vi "运维调试_五参数.vi"() -> ()   [LabVIEW 2016, in "斯坦道原位多参数.lvlib"]
uses:
  <vilib>/Utility/miscctls.llb/LVPointTypeDef.ctl
  <vilib>/Utility/config.llb/NI_LVConfig.lvlib
panel:
  in  "校准":bool
  in  "获取传感器参数并保存触发":bool
  in  "传感器参数自动获取":bool=TRUE
  in  "标样测试组数":dbl=1.0 caption="标样测试组数:"
  in  "水样测试组数":dbl=1.0 caption="水样测试组数:"
  in  "转刷清洗时间":dbl=30.0 caption="转刷清洗时间:"
  in  "上电初始化时间":dbl=5.0 caption="上电初始化时间:"
  in  "水样稳定时间":dbl=5.0 caption="水样稳定时间:"
  out "串口号":string
  in  "水深写入":bool
  in  "水深读取":bool
  in  "水深校准":dbl caption="水深校准:"
  out "模块版本号":string
  in  "写入":bool
  in  "读取":bool
  in  "B":dbl caption="校准值B:"
  in  "K":dbl caption="校准值K:"
  in  "标样核查":bool
  in  "串口设置":bool
  in  "质控参数设置":bool
  in  "打开串口":bool
  in  "释放串口":bool
  out "多参数横条运行状态":T1(xcontrol)
  in  "数据区":i32(listbox)
  in  "停止测量(单探)":bool
  in  "启动测量(单探)":bool
  in  "控制命令区探头选择":u16(ring)=9 items=["氨氮"=3, "水温"=9, "pH值"=10, "溶解氧"=11, "电导率"=12, "浊度"=13, "叶绿素a"=14, "藻密度"=15, "蓝绿藻"=16, "氧化还原电位"=17, "溶解氧%"=18, "盐度"=19]
  in  "同步时间":bool
  in  "初始化(清洗)":bool
  in  "停止测量(全部)":bool
  in  "启动测量(全部)":bool
  in  "关键参数区读取":bool
  in  "关键参数区":i32(listbox)
  in  "传感器参数读取":bool
  in  "传感器区":i32(listbox)
  in  "返回":bool
  in  "设置":bool
  out "运行状态":string
  in  "停止":bool
  in  "水样测试":bool
  out "集成报警信息":string
  # "min"
  # "组"
  # "组"
  # "s"
  # "s"
  # "控制命令区"
  # "探头校准"
  # "水深校准"
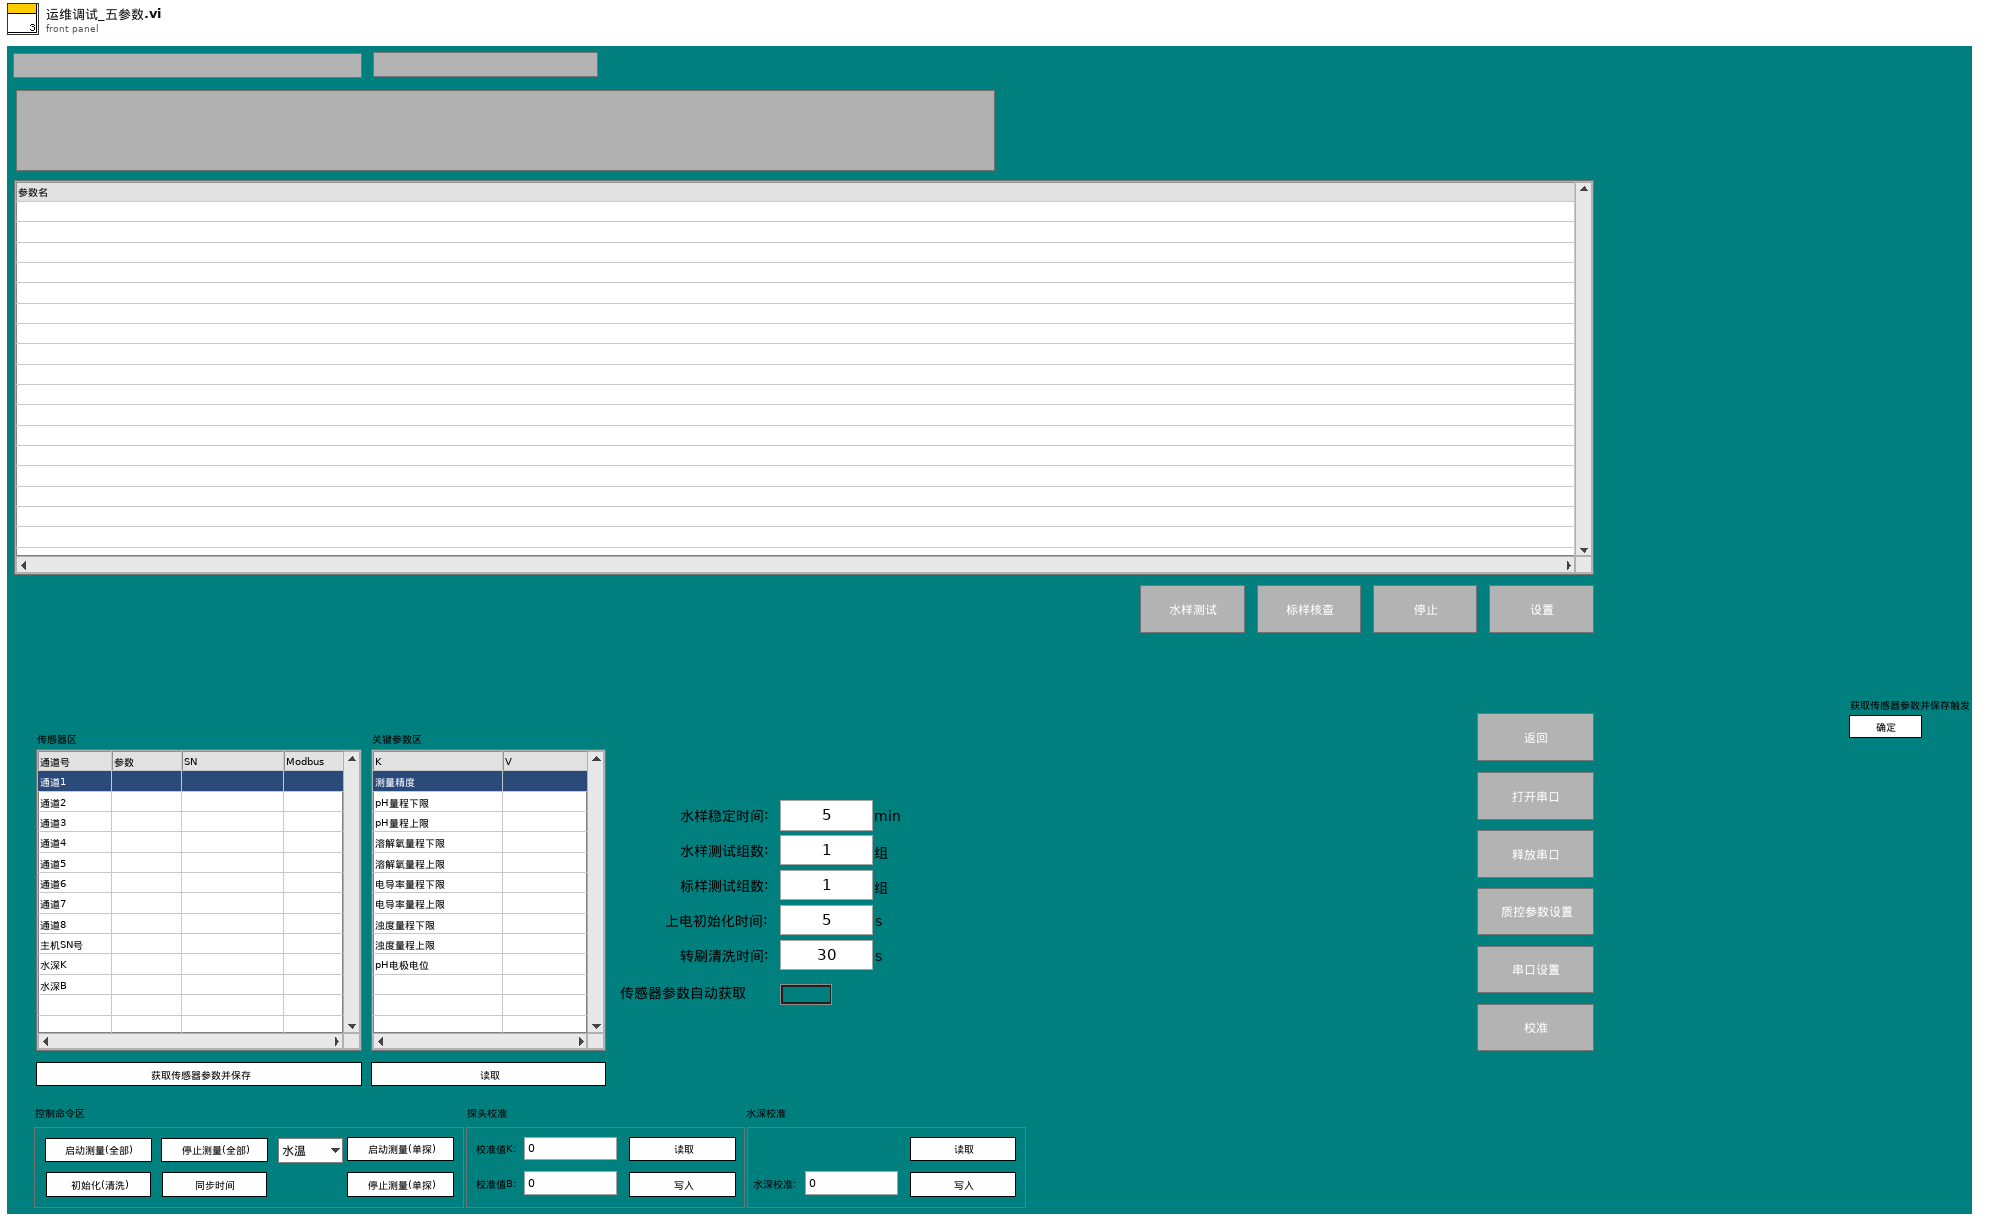
[diagram p1: front panel]
types:
  T1 = cluster{"系统时间":timestamp, "工作状态":u16, "测量模式":u16, "告警代码":enum16{"无告警", "缺试剂告警", "缺水样告警", "缺蒸馏水告警", "缺标液告警", "仪表漏液告警", "标定异常告警", "超量程告警", "加热异常", "低试剂预警", "超上限告警", "超下限告警", "仪表内部其他异常", "滴定异常告警", "电极异常告警", "量程切换告警", "参数设置告警", "PH电极电位异常", "电导率电极异常", "浊度光度异常", "溶解氧电极异常", "溶解氧光强异常", "温度异常告警", "PH异常告警", "溶解氧异常告警", "电导率异常告警", "浊度异常告警", "叶绿素异常告警", "藻密度异常告警", "蓝绿藻异常告警", "ORP异常告警", "氨氮异常告警", "清洁刷异常告警", "SD卡异常告警", "蓝牙异常告警", "Wifi异常告警", "流程异常告警"}, "故障代码":enum16{"无故障", "电机故障", "温度故障", "通讯故障", "滴定故障"}, "日志代码":u16, "软件版本":string}
  T2 = typedef "LVPointTypeDef.ctl" = cluster{"Horizontal":i16, "Vertical":i16}
  T3 = typedef "报警信息字段定义.ctl" = cluster{"时间":timestamp, "参数":string, "报警信息":string, "备注":string, "code":u64, "platform_alarm_code":string}
  T4 = enum16{"无告警", "缺试剂告警", "缺水样告警", "缺蒸馏水告警", "缺标液告警", "仪表漏液告警", "标定异常告警", "超量程告警", "加热异常", "低试剂预警", "超上限告警", "超下限告警", "仪表内部其他异常", "滴定异常告警", "电极异常告警", "量程切换告警", "参数设置告警", "PH电极电位异常", "电导率电极异常", "浊度光度异常", "溶解氧电极异常", "溶解氧光强异常", "温度异常告警", "PH异常告警", "溶解氧异常告警", "电导率异常告警", "浊度异常告警", "叶绿素异常告警", "藻密度异常告警", "蓝绿藻异常告警", "ORP异常告警", "氨氮异常告警", "清洁刷异常告警", "SD卡异常告警", "蓝牙异常告警", "Wifi异常告警", "流程异常告警"}
  T5 = cluster{"水温":dbl, "pH":dbl, "DO":dbl, "Cond":dbl, "Turb":dbl, "叶绿素":dbl, "藻密度":dbl, "蓝绿藻":dbl, "ORP":dbl, "NH3N":dbl}
  T6 = cluster{"因子编码":string, "单位":string, "标样参考值":sgl, "水样数据时间":timestamp, "水样实测值":sgl, "水样数据标识":string, "K":sgl, "B":sgl, "T":sgl, "H":sgl, "水深":sgl, "探头温度":sgl, "信号值":sgl}
  T7 = cluster{"Major":u16, "Minor":u16, "Fix":u16, "Build":u16}
  T8 = enum8{"Enabled", "Disabled", "Disabled and Grayed Out"}
  T9 = typedef "斯坦道原位多参数.lvlib/水样测试启动自定义输入参数.ctl" = cluster{"测量模式":string, "数据类型":string}
  T10 = typedef "斯坦道原位多参数.lvlib/标样核查启动自定义输入参数.ctl" = cluster{"测量模式":string, "数据类型":string, "输出参数":cluster{"水温":bool, "pH":bool, "DO":bool, "浊度":bool, "电导率":bool}}
  T11 = typedef "NI_LVConfig.lvlib/Config Data RefNum.ctl" = refnum<k1>
  T12 = cluster{"水温标准液标准浓度":dbl, "酸碱度标准液标准浓度":dbl, "溶解氧标准液标准浓度":dbl, "电导率标准液标准浓度":dbl, "浊度标准液标准浓度":dbl}
  T13 = cluster{"确定":bool, "水温标准液标准浓度":dbl, "酸碱度标准液标准浓度":dbl, "溶解氧标准液标准浓度":dbl, "电导率标准液标准浓度":dbl, "浊度标准液标准浓度":dbl}
  T14 = cluster{"运行模式":enum16{"维护模式", "常规模式", "应急模式", "质控模式"}, "24H周期设置":bool[]}
  T15 = cluster{"水温":bool, "pH":bool, "DO":bool, "浊度":bool, "电导率":bool}
  T16 = enum32{"Bad", "Idle", "Run top level", "Running"}
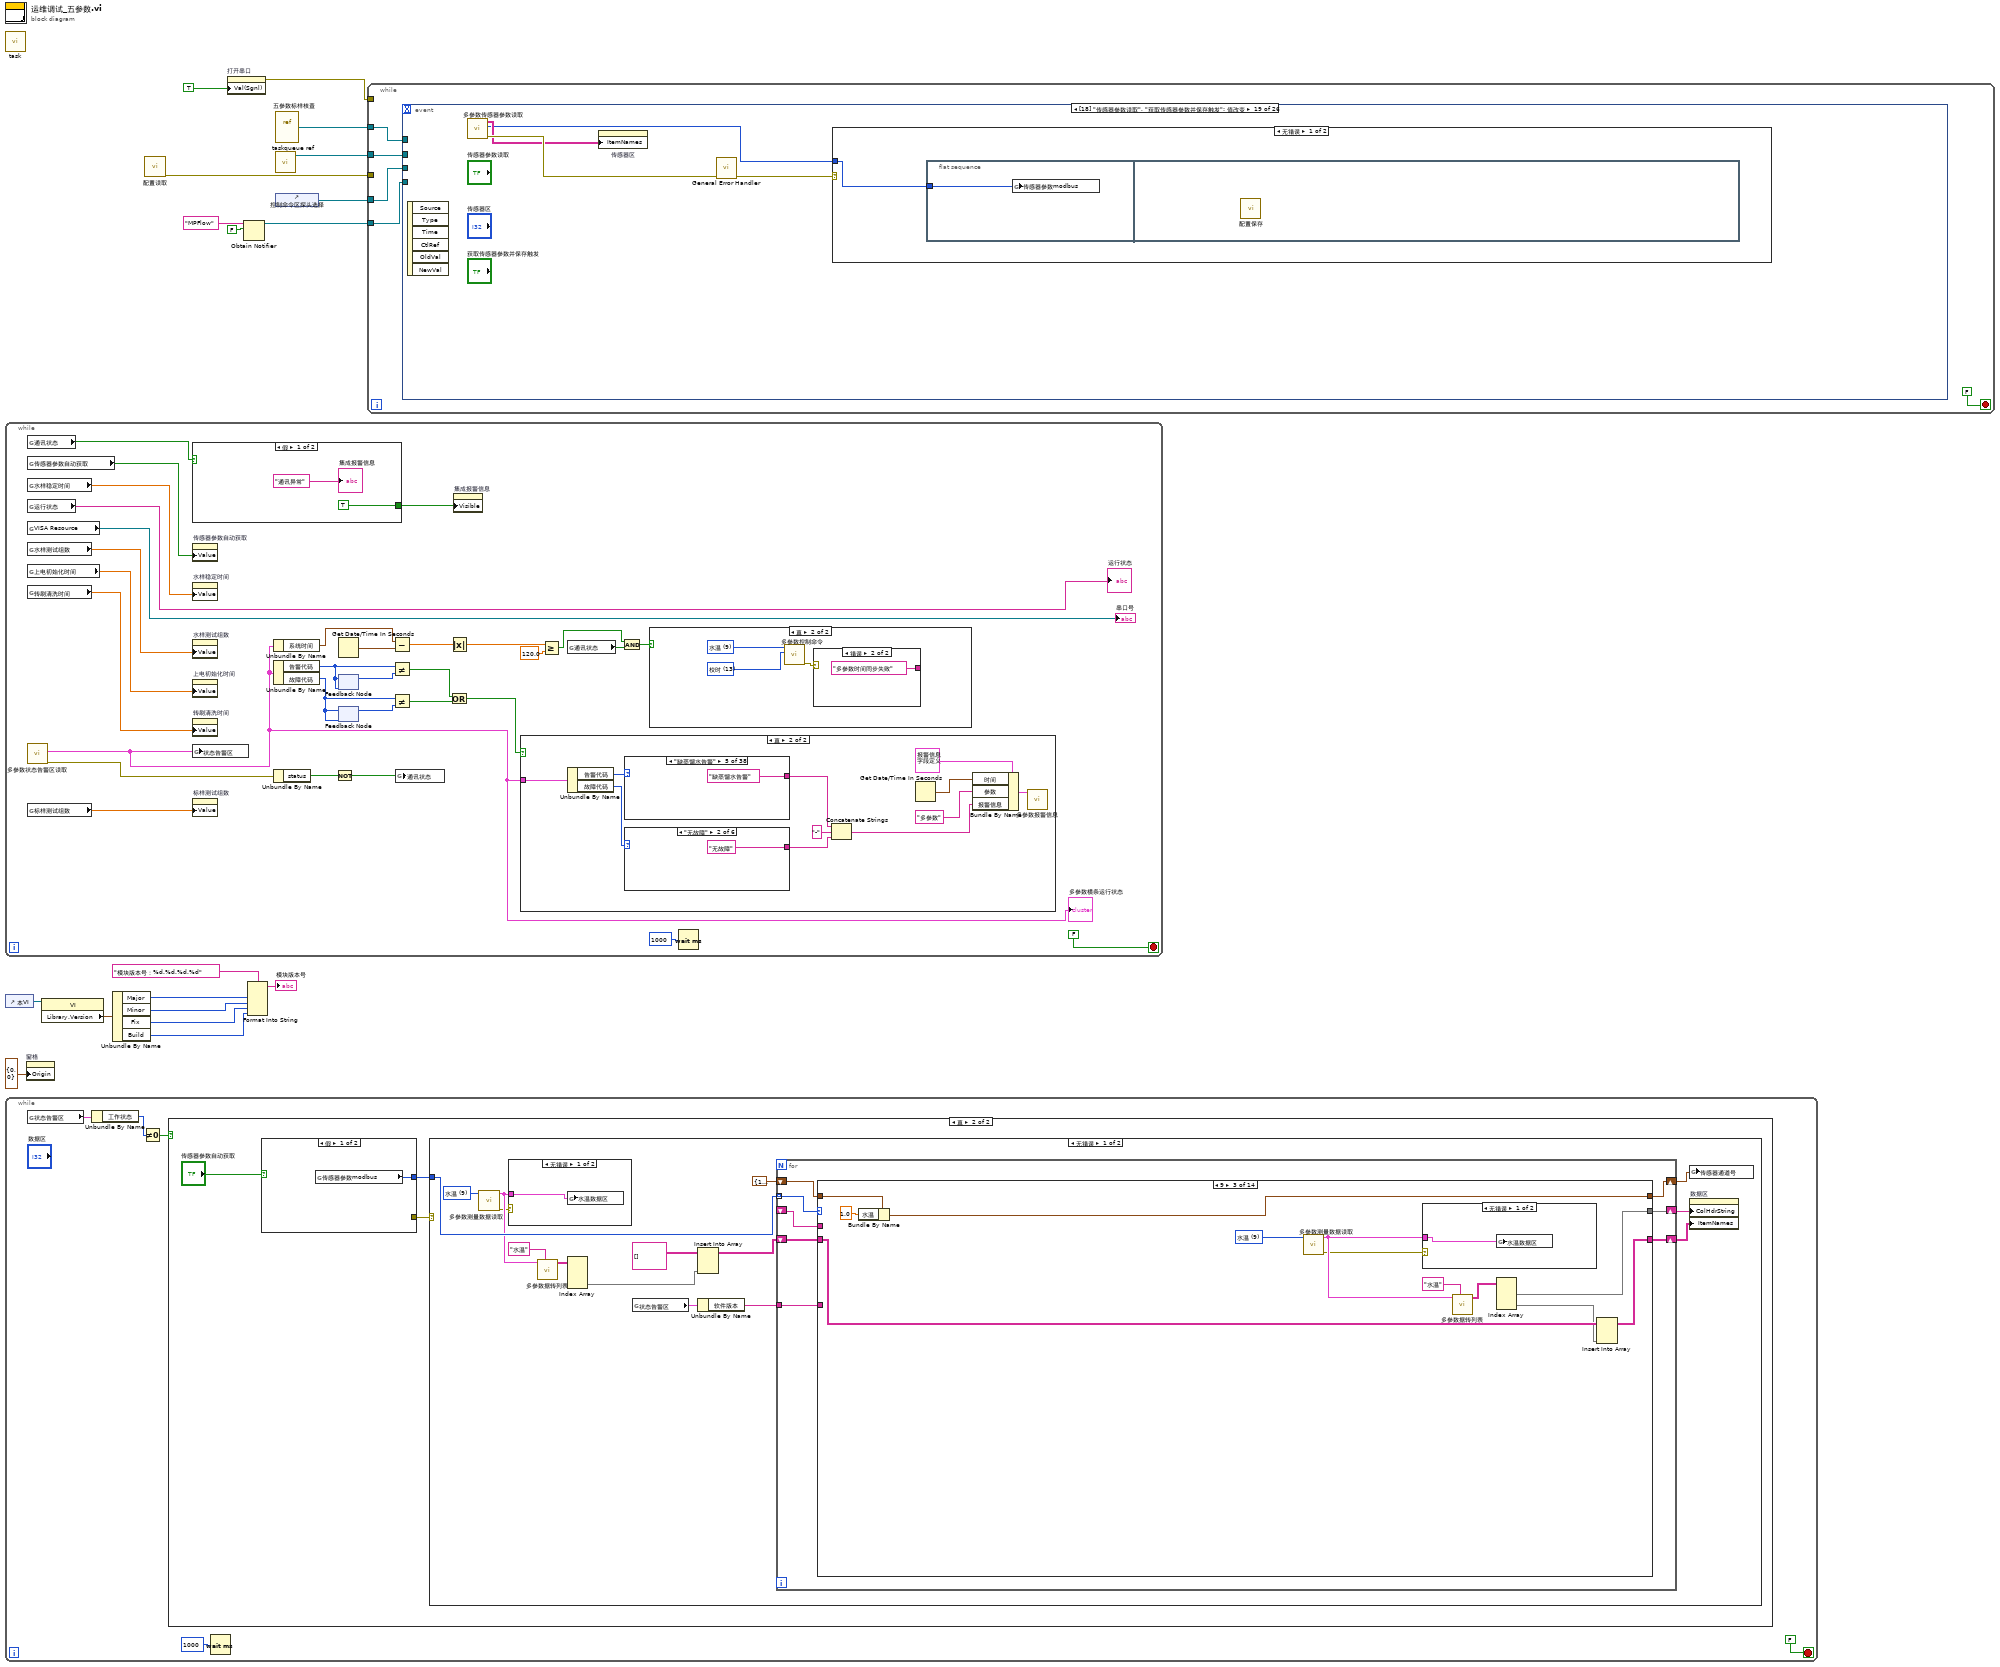
[diagram p0: block diagram]
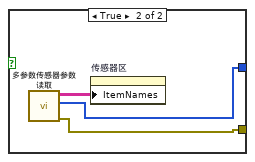
[diagram p3: hidden frame]
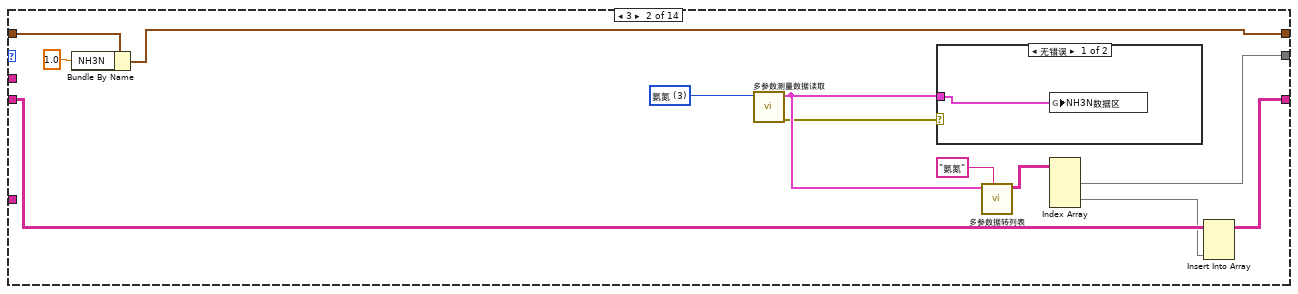
[diagram p6: hidden frame]
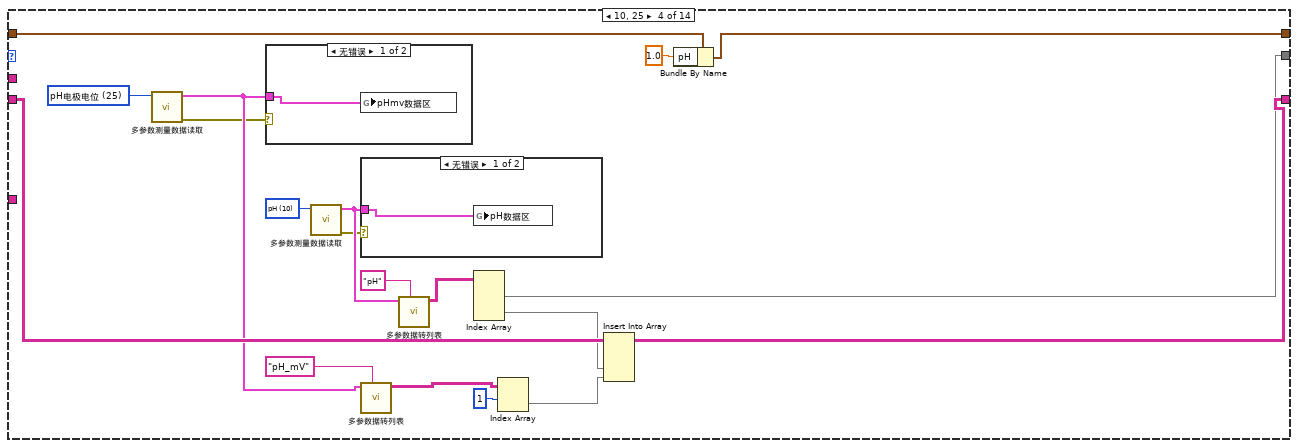
[diagram p9: hidden frame]
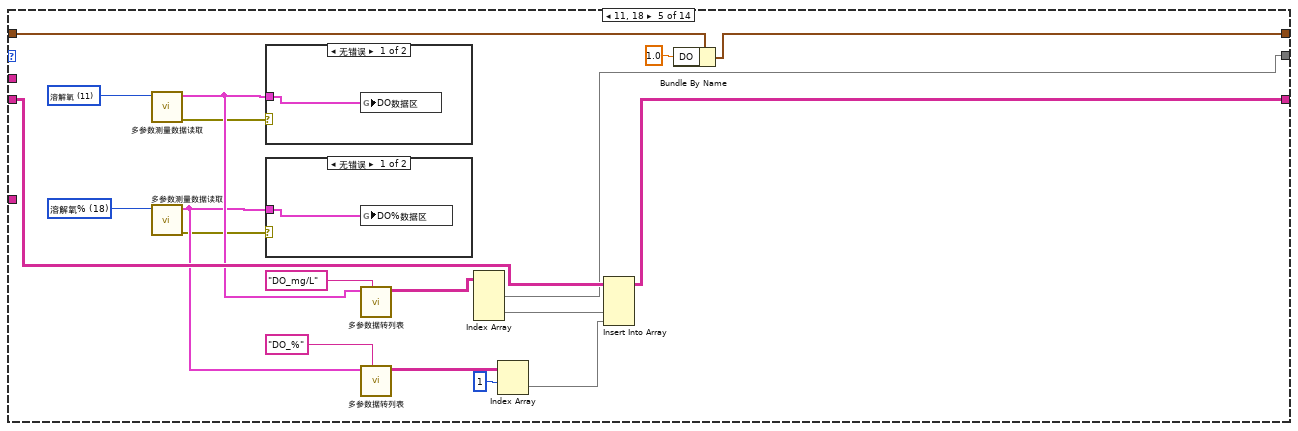
[diagram p12: hidden frame]
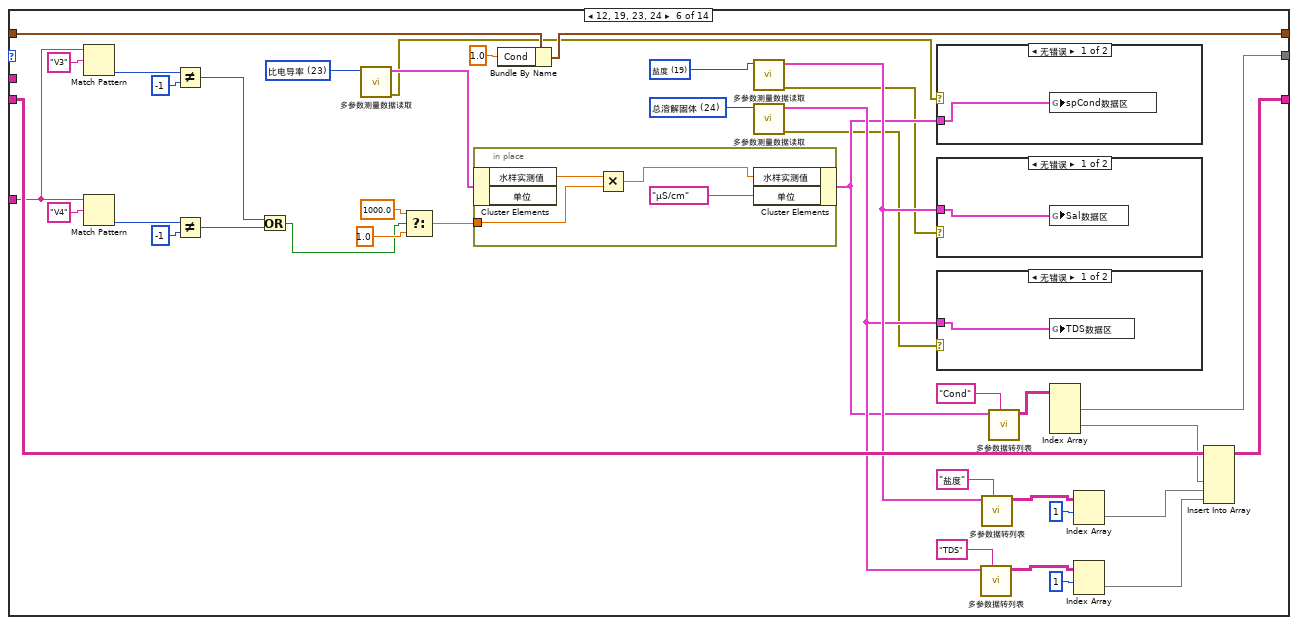
[diagram p15: hidden frame]
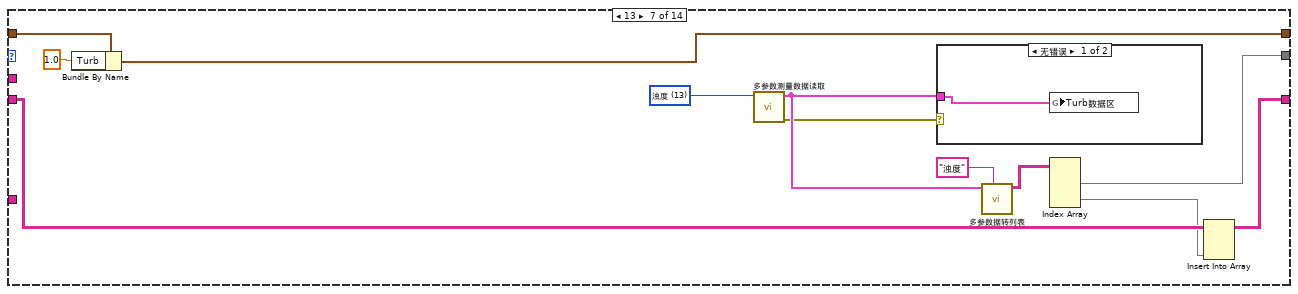
[diagram p19: hidden frame]
diagram:
  n1 = call "task.vi"() -> ()  [unwired: 12 in]
  n2 = while {
    stop <- FALSE stop-if-true
    n3 = global read "多参数全局变量.vi" "通讯状态"() -> (w47:bool)
    n4 = global read "多参数断电保存全局变量.vi" "传感器参数自动获取"() -> (w19:bool)
    n5 = global read "多参数断电保存全局变量.vi" "水样稳定时间"() -> (w24:dbl)
    n6 = global read "多参数全局变量.vi" "运行状态"() -> (→"运行状态":string)
    n7 = global read "多参数断电保存全局变量.vi" "VISA Resource"() -> (→"串口号":refnum<visa-resource-name>)
    n8 = global read "多参数断电保存全局变量.vi" "水样测试组数"() -> (w23:dbl)
    n9 = global read "多参数断电保存全局变量.vi" "上电初始化时间"() -> (w22:dbl)
    n10 = global read "多参数断电保存全局变量.vi" "转刷清洗时间"() -> (w21:dbl)
    n11 = call "多参数状态告警区读取.vi"() -> ("error out"=w37:errorcluster, "状态告警块"=w34:T1)  [unwired: 9 in, 1 out]
    "多参数横条运行状态" <- w34
    n12 = global read "多参数断电保存全局变量.vi" "标样测试组数"() -> (w20:dbl)
    n13 = case shown="假" w47 {
      tunnel: [TRUE ("可见") _] -> w46
      frame False {
        "集成报警信息" <- "通讯异常" ("集成报警信息")
      }
      frame True {
      }
    }
    n14 = property on="传感器参数自动获取" class="Bool (严格)"("Value"=w19) -> ()  [unwired: 2 in, 2 out]
    n15 = property on="水样稳定时间" class="DigNum (严格)"("Value"=w24) -> ()  [unwired: 2 in, 2 out]
    n16 = property on="水样测试组数" class="DigNum (严格)"("Value"=w23) -> ()  [unwired: 2 in, 2 out]
    n17 = property on="上电初始化时间" class="DigNum (严格)"("Value"=w22) -> ()  [unwired: 2 in, 2 out]
    n18 = property on="转刷清洗时间" class="DigNum (严格)"("Value"=w21) -> ()  [unwired: 2 in, 2 out]
    n19 = global write "多参数全局变量.vi" "状态告警区"(w34) -> ()
    n20 = property on="标样测试组数" class="DigNum (严格)"("Value"=w20) -> ()  [unwired: 2 in, 2 out]
    n21 = Unbundle By Name(w34) -> ("系统时间"=w33:timestamp)
    n22 = Unbundle By Name(w34) -> ("告警代码"=w43:T4, "故障代码"=w41:enum16{"无故障", "电机故障", "温度故障", "通讯故障", "滴定故障"})
    n23 = Unbundle By Name(w37) -> ("status"=w36:bool)
    n24 = Not(x=w36) -> (.not. x?=w35:bool)
    n25 = Get Date/Time In Seconds() -> (seconds since 1Jan1904=w32:timestamp)
    n26 = feedback #1(w43) -> (w44:T4)
    n27 = feedback-in #1(w43) -> ()
    n28 = feedback #2(w41) -> (w42:enum16{"无故障", "电机故障", "温度故障", "通讯故障", "滴定故障"})
    n29 = feedback-in #2(w41) -> ()
    n30 = Subtract(x=w33, y=w32) -> (x-y=w31:dbl)
    n31 = Not Equal?(x=w43, y=w44) -> (x != y?=w39:bool)
    n32 = Not Equal?(x=w41, y=w42) -> (x != y?=w40:bool)
    n33 = global write "多参数全局变量.vi" "通讯状态"(w35) -> ()
    n34 = Absolute Value(x=w31) -> (abs(x)=w30:dbl)
    n35 = Or(x=w39, y=w40) -> (x .or. y?=w38:bool)
    n36 = property on="集成报警信息" class="Str"("Visible"=w46) -> ()  [unwired: 2 in, 2 out]
    n37 = case shown="真" w38 {
      tunnel: w34 -> [_ w65]
      frame False {
      }
      frame True {
        n38 = Unbundle By Name(w65) -> ("告警代码"=w64:T4, "故障代码"=w63:enum16{"无故障", "电机故障", "温度故障", "通讯故障", "滴定故障"})
        n39 = case shown="\"缺蒸馏水告警\"" w64 {
          selector: w64 -> [w76 _ _ _ _ _ _ _ _ _ _ _ _ _ _ _ _ _ _ _ _ _ _ _ _ _ _ _ _ _ _ _ _ _ _ _ _ _]
          tunnel: [w75 "无告警" "缺试剂告警" "缺水样告警" "缺蒸馏水告警" "缺标液告警" "仪表漏液告警" "标定异常告警" "超量程告警" "加热异常" "低试剂预警" "超上限告警" "超下限告警" "仪表内部其他异常" "滴定异常告警" "电极异常告警" "量程切换告警" "参数设置告警" "PH电极电位异常" "电导率电极异常" "浊度光度异常" "溶解氧电极异常" "溶解氧光强异常" "温度异常告警" "PH异常告警" "溶解氧异常告警" "电导率异常告警" "浊度异常告警" "叶绿素异常告警" "藻密度异常告警" "蓝绿藻异常告警" "ORP异常告警" "氨氮异常告警" "清洁刷异常告警" "SD卡异常告警" "蓝牙异常告警" "WiFi异常告警" "流程异常告警"] -> w62
          frame Default {
            n40 = Format Into String(format string="%d" ("格式字符串"), initial string="未知" ("工作状态"), w76) -> (resulting string=w75:string)  [unwired: 1 in, 1 out]
          }
          frame "无告警" {
          }
          frame "缺试剂告警" {
          }
          frame "缺水样告警" {
          }
          frame "缺蒸馏水告警" {
          }
          frame "缺标液告警" {
          }
          frame "仪表漏液告警" {
          }
          frame "标定异常告警" {
          }
          frame "超量程告警" {
          }
          frame "加热异常" {
          }
          frame "低试剂预警" {
          }
          frame "超上限告警" {
          }
          frame "超下限告警" {
          }
          frame "仪表内部其他异常" {
          }
          frame "滴定异常告警" {
          }
          frame "电极异常告警" {
          }
          frame "量程切换告警" {
          }
          frame "参数设置告警" {
          }
          frame "PH电极电位异常" {
          }
          frame "电导率电极异常" {
          }
          frame "浊度光度异常" {
          }
          frame "溶解氧电极异常" {
          }
          frame "溶解氧光强异常" {
          }
          frame "温度异常告警" {
          }
          frame "PH异常告警" {
          }
          frame "溶解氧异常告警" {
          }
          frame "电导率异常告警" {
          }
          frame "浊度异常告警" {
          }
          frame "叶绿素异常告警" {
          }
          frame "藻密度异常告警" {
          }
          frame "蓝绿藻异常告警" {
          }
          frame "ORP异常告警" {
          }
          frame "氨氮异常告警" {
          }
          frame "清洁刷异常告警" {
          }
          frame "SD卡异常告警" {
          }
          frame "蓝牙异常告警" {
          }
          frame "Wifi异常告警" {
          }
          frame "流程异常告警" {
          }
        }
        n41 = case shown="\"无故障\"" w63 {
          selector: w63 -> [w67 _ _ _ _ _]
          tunnel: [w66 "无故障" "电机故障" "温度故障" "通讯故障" "滴定故障"] -> w61
          frame Default {
            n42 = Format Into String(format string="%d" ("格式字符串"), initial string="未知" ("工作状态"), w67) -> (resulting string=w66:string)  [unwired: 1 in, 1 out]
          }
          frame "无故障" {
          }
          frame "电机故障" {
          }
          frame "温度故障" {
          }
          frame "通讯故障" {
          }
          frame "滴定故障" {
          }
        }
        n43 = Concatenate Strings(w62, "-" ("字符串"), w61) -> (w59:string)
        n44 = Get Date/Time In Seconds() -> (seconds since 1Jan1904=w58:timestamp)
        n45 = Bundle By Name(cluster=T3 {"时间"=timestamp(0 s since 1904-01-01), "参数"="", "报警信息"="", "备注"="", "code"=0, "platform_alarm_code"=""} ("data"), "时间"=w58, "参数"="多参数" ("设备"), "报警信息"=w59) -> (w55:T3)
        n46 = call "多参数报警信息.vi"("data"=w55) -> ()  [unwired: 10 in, 1 out]
      }
    }
    n47 = Greater Or Equal?(x=w30, y=120.0) -> (x >= y?=w29:bool)
    n48 = global read "多参数全局变量.vi" "通讯状态"() -> (w26:bool)
    n49 = And(x=w29, y=w26) -> (x .and. y?=w27:bool)
    n50 = case shown="真" w27 {
      frame False {
      }
      frame True {
        w50 = u16 13 items=["启动测量（全部）"=1, "初始化（清洗）"=10, "停止测量（全部）"=11, "校时"=13, "启动测量（单个传感器）"=19, "停止测量（单个传感器）"=20] ("控制命令")
        w51 = u16 9 items=["氨氮"=3, "水温"=9, "pH值"=10, "溶解氧"=11, "电导率"=12, "浊度"=13, "叶绿素a"=14, "藻密度"=15, "蓝绿藻"=16, "氧化还原电位"=17, "溶解氧%"=18, "盐度"=19] ("站号")
        n51 = call "多参数控制命令.vi"("控制命令"=w50, "站号"=w51) -> ("error out"=w52:errorcluster)  [unwired: 9 in]
        n52 = case shown="错误" w52 {
          tunnel: ["多参数时间同步成功" ("消息") "多参数时间同步失败" ("消息")] -> _
          frame No Error {
          }
          frame Error {
          }
        }
      }
    }
    n53 = Wait (ms)(milliseconds to wait=u32 1000 ("等待时间（毫秒）")) -> ()  [unwired: 1 out]
  }
  n54 = control-ref of="本VI"() -> (w10:refnum<vi>)
  n55 = while {
    stop <- FALSE stop-if-true
    n56 = global read "多参数全局变量.vi" "状态告警区"() -> (w120:T1)
    n57 = Unbundle By Name(w120) -> ("工作状态"=w119:u16)
    n58 = Not Equal To 0?(x=w119) -> (x != 0?=w118:bool)
    n59 = case shown="真" w118 {
      frame False {
      }
      frame True {
        n60 = case shown="假" "传感器参数自动获取" {
          tunnel: [_ w129] -> w125
          tunnel: [w126 w128] -> w124
          frame False {
            n61 = global read "多参数断电保存全局变量.vi" "传感器参数modbus"() -> (w126:u16[])
          }
          frame True {
            n62 = call "多参数传感器参数读取.vi"() -> ("error out"=w129:errorcluster, "modbus"=w128:u16[], "添加的数组"=w127:string[][])  [unwired: 9 in]
            n63 = property on="传感器区" class="MCListbox (严格)"("ItemNames"=w127) -> ()  [unwired: 2 in, 2 out]
          }
        }
        n64 = case shown="无错误" w125 {
          tunnel: w124 -> [w144 _]
          frame No Error {
            w141 = u16 9 items=["氨氮"=3, "水温"=9, "pH"=10, "溶解氧"=11, "电导率"=12, "浊度"=13, "叶绿素a"=14, "藻密度"=15, "蓝绿藻"=16, "氧化还原电位"=17, "溶解氧%"=18, "盐度"=19, "水中油"=20, "高锰酸盐指数"=21, "化学需氧量"=22, "比电导率"=23, "总溶解固体"=24, "pH电极电位"=25] ("下拉列表")
            n65 = call "多参数测量数据读取.vi"("探头选择"=w141) -> ("error out"=w130:errorcluster, "测量数据块"=w136:T6)  [unwired: 8 in, 1 out]
            n66 = case shown="无错误" w130 {
              tunnel: w136 -> [w145 _]
              frame No Error {
                n67 = global write "多参数全局变量.vi" "水温数据区"(w145) -> ()
              }
              frame Error {
              }
            }
            n68 = call "多参数据转列表.vi"("参数名"="水温", "测量数据块"=w136) -> ("添加的数组"=w134:string[][])  [unwired: 9 in]
            n69 = Index Array(array=w134) -> (element #2=w133:string[])  [unwired: 4 in, 1 out]
            n70 = global read "多参数全局变量.vi" "状态告警区"() -> (w132:T1)
            n71 = Insert Into Array(array=string[][] [] ("子数组"), new element=w133) -> (w139:string[][])  [unwired: 2 in]
            n72 = Unbundle By Name(w132) -> ("软件版本"=w131:string)
            n73 = for {
              tunnel: w144 -> [w153] mode=indexing
              shift-right: [w151] -> w142
              shift-left: w139 -> [w152]
              shift-right: [w150] -> w143
              shift-left: _ -> [w149]
              shift-right: [w148] -> w137
              shift-left: T5 {"水温"=1.0, "pH"=0.0, "DO"=0.0, "Cond"=0.0, "Turb"=0.0, "叶绿素"=0.0, "藻密度"=0.0, "蓝绿藻"=0.0, "ORP"=0.0, "NH3N"=0.0} ("传感器通道号") -> [w147]
              tunnel: w131 -> [w146]
              n74 = case shown="9" w153 {
                tunnel: w152 -> [w156 w167 w180 w200 w221 w263 w282 w295 w308 w321 w334 w344 w353 w362]
                tunnel: [w156 w166 w179 w199 w220 w262 w281 w294 w307 w320 w333 w343 w352 w361] -> w151
                tunnel: [w155 w159 w172 w192 w213 w254 w275 w287 w302 w314 w327 w338 w347 w356] -> w150
                tunnel: w149 -> [w155 _ _ _ _ _ _ _ _ _ _ _ _ _]
                tunnel: [w154 w163 w176 w195 w217 w257 w278 w291 w304 w317 w330 w342 w351 w360] -> w148
                tunnel: w147 -> [w154 w165 w178 w197 w219 w258 w279 w292 w305 w318 w331 w342 w351 w360]
                tunnel: w146 -> [_ _ _ _ _ w233 _ _ _ _ _ _ _ _]
                frame 0, Default {
                }
                frame 3 {
                  w168 = u16 3 items=["氨氮"=3, "水温"=9, "pH"=10, "溶解氧"=11, "电导率"=12, "浊度"=13, "叶绿素a"=14, "藻密度"=15, "蓝绿藻"=16, "氧化还原电位"=17, "溶解氧%"=18, "盐度"=19, "水中油"=20, "高锰酸盐指数"=21, "化学需氧量"=22, "比电导率"=23, "总溶解固体"=24, "pH电极电位"=25] ("下拉列表")
                  n75 = Bundle By Name(cluster=w165, "NH3N"=1.0) -> (w163:T5)
                  n76 = call "多参数测量数据读取.vi"("探头选择"=w168) -> ("error out"=w157:errorcluster, "测量数据块"=w162:T6)  [unwired: 8 in, 1 out]
                  n77 = case shown="无错误" w157 {
                    tunnel: w162 -> [w169 _]
                    frame No Error {
                      n78 = global write "多参数全局变量.vi" "NH3N数据区"(w169) -> ()
                    }
                    frame Error {
                    }
                  }
                  n79 = call "多参数据转列表.vi"("参数名"="氨氮", "测量数据块"=w162) -> ("添加的数组"=w161:string[][])  [unwired: 9 in]
                  n80 = Index Array(array=w161) -> (element #1=w159:string[], element #2=w158:string[])  [unwired: 4 in]
                  n81 = Insert Into Array(array=w167, new element=w158) -> (w166:string[][])  [unwired: 2 in]
                }
                frame 9 {
                  w181 = u16 9 items=["氨氮"=3, "水温"=9, "pH"=10, "溶解氧"=11, "电导率"=12, "浊度"=13, "叶绿素a"=14, "藻密度"=15, "蓝绿藻"=16, "氧化还原电位"=17, "溶解氧%"=18, "盐度"=19, "水中油"=20, "高锰酸盐指数"=21, "化学需氧量"=22, "比电导率"=23, "总溶解固体"=24, "pH电极电位"=25] ("下拉列表")
                  n82 = Bundle By Name(cluster=w178, "水温"=1.0) -> (w176:T5)
                  n83 = call "多参数测量数据读取.vi"("探头选择"=w181) -> ("error out"=w170:errorcluster, "测量数据块"=w175:T6)  [unwired: 8 in, 1 out]
                  n84 = case shown="无错误" w170 {
                    tunnel: w175 -> [w182 _]
                    frame No Error {
                      n85 = global write "多参数全局变量.vi" "水温数据区"(w182) -> ()
                    }
                    frame Error {
                    }
                  }
                  n86 = call "多参数据转列表.vi"("参数名"="水温", "测量数据块"=w175) -> ("添加的数组"=w174:string[][])  [unwired: 9 in]
                  n87 = Index Array(array=w174) -> (element #1=w172:string[], element #2=w171:string[])  [unwired: 4 in]
                  n88 = Insert Into Array(array=w180, new element=w171) -> (w179:string[][])  [unwired: 2 in]
                }
                frame 10, 25 {
                  w198 = u16 25 items=["氨氮"=3, "水温"=9, "pH"=10, "溶解氧"=11, "电导率"=12, "浊度"=13, "叶绿素a"=14, "藻密度"=15, "蓝绿藻"=16, "氧化还原电位"=17, "溶解氧%"=18, "盐度"=19, "水中油"=20, "高锰酸盐指数"=21, "化学需氧量"=22, "比电导率"=23, "总溶解固体"=24, "pH电极电位"=25] ("下拉列表")
                  w201 = u16 10 items=["氨氮"=3, "水温"=9, "pH"=10, "溶解氧"=11, "电导率"=12, "浊度"=13, "叶绿素a"=14, "藻密度"=15, "蓝绿藻"=16, "氧化还原电位"=17, "溶解氧%"=18, "盐度"=19, "水中油"=20, "高锰酸盐指数"=21, "化学需氧量"=22, "比电导率"=23, "总溶解固体"=24, "pH电极电位"=25] ("下拉列表")
                  n89 = call "多参数测量数据读取.vi"("探头选择"=w198) -> ("error out"=w183:errorcluster, "测量数据块"=w188:T6)  [unwired: 8 in, 1 out]
                  n90 = case shown="无错误" w183 {
                    tunnel: w188 -> [w202 _]
                    frame No Error {
                      n91 = global write "多参数全局变量.vi" "pHmv数据区"(w202) -> ()
                    }
                    frame Error {
                    }
                  }
                  n92 = call "多参数测量数据读取.vi"("探头选择"=w201) -> ("error out"=w184:errorcluster, "测量数据块"=w194:T6)  [unwired: 8 in, 1 out]
                  n93 = case shown="无错误" w184 {
                    tunnel: w194 -> [w203 _]
                    frame No Error {
                      n94 = global write "多参数全局变量.vi" "pH数据区"(w203) -> ()
                    }
                    frame Error {
                    }
                  }
                  n95 = call "多参数据转列表.vi"("参数名"="pH_mV", "测量数据块"=w188) -> ("添加的数组"=w187:string[][])  [unwired: 9 in]
                  n96 = call "多参数据转列表.vi"("参数名"="pH", "测量数据块"=w194) -> ("添加的数组"=w193:string[][])  [unwired: 9 in]
                  n97 = Index Array(array=w193) -> (element #1=w192:string[], element #2=w191:string[])  [unwired: 4 in]
                  n98 = Index Array(array=w187, index (row)=1 ("禁用的索引 (列)")) -> (element=w190:string[])  [unwired: 1 in]
                  n99 = Insert Into Array(array=w200, new element #1=w191, new element #2=w190) -> (w199:string[][])  [unwired: 2 in]
                  n100 = Bundle By Name(cluster=w197, "pH"=1.0) -> (w195:T5)
                }
                frame 11, 18 {
                  w211 = u16 18 items=["氨氮"=3, "水温"=9, "pH"=10, "溶解氧"=11, "电导率"=12, "浊度"=13, "叶绿素a"=14, "藻密度"=15, "蓝绿藻"=16, "氧化还原电位"=17, "溶解氧%"=18, "盐度"=19, "水中油"=20, "高锰酸盐指数"=21, "化学需氧量"=22, "比电导率"=23, "总溶解固体"=24, "pH电极电位"=25] ("下拉列表")
                  w222 = u16 11 items=["氨氮"=3, "水温"=9, "pH"=10, "溶解氧"=11, "电导率"=12, "浊度"=13, "叶绿素a"=14, "藻密度"=15, "蓝绿藻"=16, "氧化还原电位"=17, "溶解氧%"=18, "盐度"=19, "水中油"=20, "高锰酸盐指数"=21, "化学需氧量"=22, "比电导率"=23, "总溶解固体"=24, "pH电极电位"=25] ("下拉列表")
                  n101 = call "多参数测量数据读取.vi"("探头选择"=w222) -> ("error out"=w205:errorcluster, "测量数据块"=w216:T6)  [unwired: 8 in, 1 out]
                  n102 = call "多参数测量数据读取.vi"("探头选择"=w211) -> ("error out"=w204:errorcluster, "测量数据块"=w210:T6)  [unwired: 8 in, 1 out]
                  n103 = case shown="无错误" w205 {
                    tunnel: w216 -> [w224 _]
                    frame No Error {
                      n104 = global write "多参数全局变量.vi" "DO数据区"(w224) -> ()
                    }
                    frame Error {
                    }
                  }
                  n105 = case shown="无错误" w204 {
                    tunnel: w210 -> [w223 _]
                    frame No Error {
                      n106 = global write "多参数全局变量.vi" "DO%数据区"(w223) -> ()
                    }
                    frame Error {
                    }
                  }
                  n107 = call "多参数据转列表.vi"("参数名"="DO_mg/L", "测量数据块"=w216) -> ("添加的数组"=w214:string[][])  [unwired: 9 in]
                  n108 = call "多参数据转列表.vi"("参数名"="DO_%", "测量数据块"=w210) -> ("添加的数组"=w208:string[][])  [unwired: 9 in]
                  n109 = Index Array(array=w214) -> (element #1=w213:string[], element #2=w212:string[])  [unwired: 4 in]
                  n110 = Index Array(array=w208, index (row)=1 ("禁用的索引 (列)")) -> (element=w207:string[])  [unwired: 1 in]
                  n111 = Insert Into Array(array=w221, new element #1=w212, new element #2=w207) -> (w220:string[][])  [unwired: 2 in]
                  n112 = Bundle By Name(cluster=w219, "DO"=1.0) -> (w217:T5)
                }
                frame 12, 19, 23, 24 {
                  w260 = u16 24 items=["氨氮"=3, "水温"=9, "pH"=10, "溶解氧"=11, "电导率"=12, "浊度"=13, "叶绿素a"=14, "藻密度"=15, "蓝绿藻"=16, "氧化还原电位"=17, "溶解氧%"=18, "盐度"=19, "水中油"=20, "高锰酸盐指数"=21, "化学需氧量"=22, "比电导率"=23, "总溶解固体"=24, "pH电极电位"=25] ("下拉列表")
                  w261 = u16 19 items=["氨氮"=3, "水温"=9, "pH"=10, "溶解氧"=11, "电导率"=12, "浊度"=13, "叶绿素a"=14, "藻密度"=15, "蓝绿藻"=16, "氧化还原电位"=17, "溶解氧%"=18, "盐度"=19, "水中油"=20, "高锰酸盐指数"=21, "化学需氧量"=22, "比电导率"=23, "总溶解固体"=24, "pH电极电位"=25] ("下拉列表")
                  w264 = u16 23 items=["氨氮"=3, "水温"=9, "pH"=10, "溶解氧"=11, "电导率"=12, "浊度"=13, "叶绿素a"=14, "藻密度"=15, "蓝绿藻"=16, "氧化还原电位"=17, "溶解氧%"=18, "盐度"=19, "水中油"=20, "高锰酸盐指数"=21, "化学需氧量"=22, "比电导率"=23, "总溶解固体"=24, "pH电极电位"=25] ("下拉列表")
                  n113 = Match Pattern(string=w233, regular expression="V3" ("正则表达式")) -> (offset past match=w241:i32)  [unwired: 1 in, 3 out]
                  n114 = Match Pattern(string=w233, regular expression="V4" ("正则表达式")) -> (offset past match=w235:i32)  [unwired: 1 in, 3 out]
                  n115 = Not Equal?(x=w241, y=-1) -> (x != y?=w231:bool)
                  n116 = Not Equal?(x=w235, y=-1) -> (x != y?=w232:bool)
                  n117 = Or(x=w231, y=w232) -> (x .or. y?=w230:bool)
                  n118 = call "多参数测量数据读取.vi"("探头选择"=w264) -> ("error out"=w227:errorcluster, "测量数据块"=w246:T6)  [unwired: 8 in, 1 out]
                  n119 = Select(t=1000.0, s=w230, f=1.0) -> (s? t:f=w237:dbl)
                  n120 = in-place {
                    in-place-border: w237 -> [w268]
                    n121 = in-place-cluster #3(w246) -> ("水样实测值"=w270:sgl)  [unwired: 1 out]
                    n122 = Multiply(x=w270, y=w268) -> (x*y=w269:dbl)
                    n123 = in-place-cluster #3("水样实测值"=w269, "单位"="μS/cm") -> (w245:T6)
                  }
                  n124 = Bundle By Name(cluster=w258, "Cond"=1.0 ("DO")) -> (w257:T5)
                  n125 = call "多参数测量数据读取.vi"("探头选择"=w261) -> ("error out"=w226:errorcluster, "测量数据块"=w251:T6)  [unwired: 8 in, 1 out]
                  n126 = call "多参数测量数据读取.vi"("探头选择"=w260) -> ("error out"=w225:errorcluster, "测量数据块"=w248:T6)  [unwired: 8 in, 1 out]
                  n127 = case shown="无错误" w227 {
                    tunnel: w245 -> [w267 _]
                    frame No Error {
                      n128 = global write "多参数全局变量.vi" "spCond数据区"(w267) -> ()
                    }
                    frame Error {
                    }
                  }
                  n129 = case shown="无错误" w226 {
                    tunnel: w251 -> [w266 _]
                    frame No Error {
                      n130 = global write "多参数全局变量.vi" "Sal数据区"(w266) -> ()
                    }
                    frame Error {
                    }
                  }
                  n131 = case shown="无错误" w225 {
                    tunnel: w248 -> [w265 _]
                    frame No Error {
                      n132 = global write "多参数全局变量.vi" "TDS数据区"(w265) -> ()
                    }
                    frame Error {
                    }
                  }
                  n133 = call "多参数据转列表.vi"("参数名"="TDS", "测量数据块"=w248) -> ("添加的数组"=w247:string[][])  [unwired: 9 in]
                  n134 = call "多参数据转列表.vi"("参数名"="盐度", "测量数据块"=w251) -> ("添加的数组"=w250:string[][])  [unwired: 9 in]
                  n135 = call "多参数据转列表.vi"("参数名"="Cond", "测量数据块"=w245) -> ("添加的数组"=w255:string[][])  [unwired: 9 in]
                  n136 = Index Array(array=w255) -> (element #1=w254:string[], element #2=w253:string[])  [unwired: 4 in]
                  n137 = Index Array(array=w250, index (row)=1 ("禁用的索引 (列)")) -> (element=w229:string[])  [unwired: 1 in]
                  n138 = Index Array(array=w247, index (row)=1 ("禁用的索引 (列)")) -> (element=w228:string[])  [unwired: 1 in]
                  n139 = Insert Into Array(array=w263, new element #1=w253, new element #2=w229, new element #3=w228) -> (w262:string[][])  [unwired: 2 in]
                }
                frame 13 {
                  w283 = u16 13 items=["氨氮"=3, "水温"=9, "pH"=10, "溶解氧"=11, "电导率"=12, "浊度"=13, "叶绿素a"=14, "藻密度"=15, "蓝绿藻"=16, "氧化还原电位"=17, "溶解氧%"=18, "盐度"=19, "水中油"=20, "高锰酸盐指数"=21, "化学需氧量"=22, "比电导率"=23, "总溶解固体"=24, "pH电极电位"=25] ("下拉列表")
                  n140 = Bundle By Name(cluster=w279, "Turb"=1.0 ("DO")) -> (w278:T5)
                  n141 = call "多参数测量数据读取.vi"("探头选择"=w283) -> ("error out"=w272:errorcluster, "测量数据块"=w273:T6)  [unwired: 8 in, 1 out]
                  n142 = case shown="无错误" w272 {
                    tunnel: w273 -> [w284 _]
                    frame No Error {
                      n143 = global write "多参数全局变量.vi" "Turb数据区"(w284) -> ()
                    }
                    frame Error {
                    }
                  }
                  n144 = call "多参数据转列表.vi"("参数名"="浊度", "测量数据块"=w273) -> ("添加的数组"=w276:string[][])  [unwired: 9 in]
                  n145 = Index Array(array=w276) -> (element #1=w275:string[], element #2=w274:string[])  [unwired: 4 in]
                  n146 = Insert Into Array(array=w282, new element=w274) -> (w281:string[][])  [unwired: 2 in]
                }
                frame 14 {
                  w296 = u16 14 items=["氨氮"=3, "水温"=9, "pH"=10, "溶解氧"=11, "电导率"=12, "浊度"=13, "叶绿素a"=14, "藻密度"=15, "蓝绿藻"=16, "氧化还原电位"=17, "溶解氧%"=18, "盐度"=19, "水中油"=20, "高锰酸盐指数"=21, "化学需氧量"=22, "比电导率"=23, "总溶解固体"=24, "pH电极电位"=25] ("下拉列表")
                  n147 = Bundle By Name(cluster=w292, "叶绿素"=1.0 ("DO")) -> (w291:T5)
                  n148 = call "多参数测量数据读取.vi"("探头选择"=w296) -> ("error out"=w285:errorcluster, "测量数据块"=w290:T6)  [unwired: 8 in, 1 out]
                  n149 = case shown="无错误" w285 {
                    tunnel: w290 -> [w297 _]
                    frame No Error {
                      n150 = global write "多参数全局变量.vi" "叶绿素数据区"(w297) -> ()
                    }
                    frame Error {
                    }
                  }
                  n151 = call "多参数据转列表.vi"("参数名"="叶绿素a", "测量数据块"=w290) -> ("添加的数组"=w288:string[][])  [unwired: 9 in]
                  n152 = Index Array(array=w288) -> (element #1=w287:string[], element #2=w286:string[])  [unwired: 4 in]
                  n153 = Insert Into Array(array=w295, new element=w286) -> (w294:string[][])  [unwired: 2 in]
                }
                frame 15 {
                  w309 = u16 15 items=["氨氮"=3, "水温"=9, "pH"=10, "溶解氧"=11, "电导率"=12, "浊度"=13, "叶绿素a"=14, "藻密度"=15, "蓝绿藻"=16, "氧化还原电位"=17, "溶解氧%"=18, "盐度"=19, "水中油"=20, "高锰酸盐指数"=21, "化学需氧量"=22, "比电导率"=23, "总溶解固体"=24, "pH电极电位"=25] ("下拉列表")
                  n154 = call "多参数测量数据读取.vi"("探头选择"=w309) -> ("error out"=w298:errorcluster, "测量数据块"=w301:T6)  [unwired: 8 in, 1 out]
                  n155 = case shown="无错误" w298 {
                    tunnel: w301 -> [w310 _]
                    frame No Error {
                      n156 = global write "多参数全局变量.vi" "藻密度数据区"(w310) -> ()
                    }
                    frame Error {
                    }
                  }
                  n157 = call "多参数据转列表.vi"("参数名"="藻密度", "测量数据块"=w301) -> ("添加的数组"=w303:string[][])  [unwired: 9 in]
                  n158 = Index Array(array=w303) -> (element #1=w302:string[], element #2=w300:string[])  [unwired: 4 in]
                  n159 = Insert Into Array(array=w308, new element=w300) -> (w307:string[][])  [unwired: 2 in]
                  n160 = Bundle By Name(cluster=w305, "藻密度"=1.0 ("DO")) -> (w304:T5)
                }
                frame 16 {
                  w322 = u16 16 items=["氨氮"=3, "水温"=9, "pH"=10, "溶解氧"=11, "电导率"=12, "浊度"=13, "叶绿素a"=14, "藻密度"=15, "蓝绿藻"=16, "氧化还原电位"=17, "溶解氧%"=18, "盐度"=19, "水中油"=20, "高锰酸盐指数"=21, "化学需氧量"=22, "比电导率"=23, "总溶解固体"=24, "pH电极电位"=25] ("下拉列表")
                  n161 = call "多参数测量数据读取.vi"("探头选择"=w322) -> ("error out"=w311:errorcluster, "测量数据块"=w316:T6)  [unwired: 8 in, 1 out]
                  n162 = case shown="无错误" w311 {
                    tunnel: w316 -> [w323 _]
                    frame No Error {
                      n163 = global write "多参数全局变量.vi" "蓝绿藻数据区"(w323) -> ()
                    }
                    frame Error {
                    }
                  }
                  n164 = call "多参数据转列表.vi"("参数名"="蓝绿藻", "测量数据块"=w316) -> ("添加的数组"=w315:string[][])  [unwired: 9 in]
                  n165 = Index Array(array=w315) -> (element #1=w314:string[], element #2=w313:string[])  [unwired: 4 in]
                  n166 = Insert Into Array(array=w321, new element=w313) -> (w320:string[][])  [unwired: 2 in]
                  n167 = Bundle By Name(cluster=w318, "蓝绿藻"=1.0 ("DO")) -> (w317:T5)
                }
                frame 17 {
                  w335 = u16 17 items=["氨氮"=3, "水温"=9, "pH"=10, "溶解氧"=11, "电导率"=12, "浊度"=13, "叶绿素a"=14, "藻密度"=15, "蓝绿藻"=16, "氧化还原电位"=17, "溶解氧%"=18, "盐度"=19, "水中油"=20, "高锰酸盐指数"=21, "化学需氧量"=22, "比电导率"=23, "总溶解固体"=24, "pH电极电位"=25] ("下拉列表")
                  n168 = Bundle By Name(cluster=w331, "ORP"=1.0 ("DO")) -> (w330:T5)
                  n169 = call "多参数测量数据读取.vi"("探头选择"=w335) -> ("error out"=w324:errorcluster, "测量数据块"=w329:T6)  [unwired: 8 in, 1 out]
                  n170 = case shown="无错误" w324 {
                    tunnel: w329 -> [w336 _]
                    frame No Error {
                      n171 = global write "多参数全局变量.vi" "ORP数据区"(w336) -> ()
                    }
                    frame Error {
                    }
                  }
                  n172 = call "多参数据转列表.vi"("参数名"="ORP", "测量数据块"=w329) -> ("添加的数组"=w328:string[][])  [unwired: 9 in]
                  n173 = Index Array(array=w328) -> (element #1=w327:string[], element #2=w325:string[])  [unwired: 4 in]
                  n174 = Insert Into Array(array=w334, new element=w325) -> (w333:string[][])  [unwired: 2 in]
                }
                frame 20 {
                  w345 = u16 20 items=["氨氮"=3, "水温"=9, "pH"=10, "溶解氧"=11, "电导率"=12, "浊度"=13, "叶绿素a"=14, "藻密度"=15, "蓝绿藻"=16, "氧化还原电位"=17, "溶解氧%"=18, "盐度"=19, "水中油"=20, "高锰酸盐指数"=21, "化学需氧量"=22, "比电导率"=23, "总溶解固体"=24, "pH电极电位"=25] ("下拉列表")
                  n175 = call "多参数测量数据读取.vi"("探头选择"=w345) -> ("测量数据块"=w341:T6)  [unwired: 8 in, 2 out]
                  n176 = call "多参数据转列表.vi"("参数名"="水中油", "测量数据块"=w341) -> ("添加的数组"=w339:string[][])  [unwired: 9 in]
                  n177 = Index Array(array=w339) -> (element #1=w338:string[], element #2=w337:string[])  [unwired: 4 in]
                  n178 = Insert Into Array(array=w344, new element=w337) -> (w343:string[][])  [unwired: 2 in]
                }
                frame 21 {
                  w354 = u16 21 items=["氨氮"=3, "水温"=9, "pH"=10, "溶解氧"=11, "电导率"=12, "浊度"=13, "叶绿素a"=14, "藻密度"=15, "蓝绿藻"=16, "氧化还原电位"=17, "溶解氧%"=18, "盐度"=19, "水中油"=20, "高锰酸盐指数"=21, "化学需氧量"=22, "比电导率"=23, "总溶解固体"=24, "pH电极电位"=25] ("下拉列表")
                  n179 = call "多参数测量数据读取.vi"("探头选择"=w354) -> ("测量数据块"=w350:T6)  [unwired: 8 in, 2 out]
                  n180 = call "多参数据转列表.vi"("参数名"="高锰酸盐指数", "测量数据块"=w350) -> ("添加的数组"=w349:string[][])  [unwired: 9 in]
                  n181 = Index Array(array=w349) -> (element #1=w347:string[], element #2=w346:string[])  [unwired: 4 in]
                  n182 = Insert Into Array(array=w353, new element=w346) -> (w352:string[][])  [unwired: 2 in]
                }
                frame 22 {
                  w363 = u16 22 items=["氨氮"=3, "水温"=9, "pH"=10, "溶解氧"=11, "电导率"=12, "浊度"=13, "叶绿素a"=14, "藻密度"=15, "蓝绿藻"=16, "氧化还原电位"=17, "溶解氧%"=18, "盐度"=19, "水中油"=20, "高锰酸盐指数"=21, "化学需氧量"=22, "比电导率"=23, "总溶解固体"=24, "pH电极电位"=25] ("下拉列表")
                  n183 = call "多参数测量数据读取.vi"("探头选择"=w363) -> ("测量数据块"=w359:T6)  [unwired: 8 in, 2 out]
                  n184 = call "多参数据转列表.vi"("参数名"="化学需氧量", "测量数据块"=w359) -> ("添加的数组"=w358:string[][])  [unwired: 9 in]
                  n185 = Index Array(array=w358) -> (element #1=w356:string[], element #2=w355:string[])  [unwired: 4 in]
                  n186 = Insert Into Array(array=w362, new element=w355) -> (w361:string[][])  [unwired: 2 in]
                }
              }
            }
            n187 = global write "多参数全局变量.vi" "传感器通道号"(w137) -> ()
            n188 = property on="数据区" class="MCListbox (严格)"("ColHdrString"=w143, "ItemNames"=w142) -> ()  [unwired: 2 in, 2 out]
          }
          frame Error {
          }
        }
      }
    }
    n189 = Wait (ms)(milliseconds to wait=u32 1000 ("等待时间（毫秒）")) -> ()  [unwired: 1 out]
  }
  n190 = property on="窗格" class="Pane"("Origin"=T2 {"Horizontal"=0, "Vertical"=0} ("原点")) -> ()  [unwired: 2 in, 2 out]
  n191 = property class="VI"(reference=w10) -> ("Library.Version"=w9:T7)  [unwired: 1 in, 2 out]
  n192 = Unbundle By Name(w9) -> ("Major"=w7:u16, "Minor"=w6:u16, "Fix"=w5:u16, "Build"=w4:u16)
  n193 = call "配置读取.vi"() -> ("error out"=w1:errorcluster)  [unwired: 11 in]
  n194 = property on="打开串口" class="Bool (严格)"("Val(Sgnl)"=TRUE ("值(信号)")) -> (error out=w12:errorcluster)  [unwired: 2 in, 1 out]
  n195 = Obtain Notifier(name (unnamed)="MPFlow" ("名称（未命名）"), notification data type=FALSE) -> (notifier out=w15:refnum<notifier>)  [unwired: 2 in, 2 out]
  n196 = Format Into String(format string="模块版本号：%d.%d.%d.%d" ("格式字符串"), w7, w6, w5, w4) -> (resulting string=→"模块版本号":string)  [unwired: 2 in, 1 out]
  n197 = vi-ref "五参数标样核查.vi"() -> (w11:refnum<vi>)
  n198 = call "taskqueue ref.vi"() -> ("队列输出"=w2:refnum<queue>)  [unwired: 10 in, 1 out]
  n199 = control-ref of="控制命令区探头选择"() -> (w14:refnum<vi>)
  n200 = while {
    tunnel: w15 -> [w367]
    tunnel: w14 -> [w366]
    tunnel: w12 -> [_]
    tunnel: w11 -> [w365]
    tunnel: w2 -> [w364]
    tunnel: w1 -> [_]
    stop <- FALSE stop-if-true
    n201 = event shown="[18] \"传感器参数读取\", \"获取传感器参数并保存触发\": 值改变" {
      selector: _ -> [_ _ _ _ _ _ _ _ _ _ _ _ _ _ _ _ _ _ _ _ _ _ _ _ _ _]
      dyn-events: _ -> [_ _ _ _ _ _ _ _ _ _ _ _ _ _ _ _ _ _ _ _ _ _ _ _ _ _]
      timeout: _ -> [_ _ _ _ _ _ _ _ _ _ _ _ _ _ _ _ _ _ _ _ _ _ _ _ _ _]
      tunnel: w367 -> [_ _ _ _ _ _ _ _ _ _ _ _ _ _ _ w505 _ _ _ _ _ _ _ _ _ _]
      tunnel: w366 -> [_ _ _ w376 w380 _ _ _ _ _ _ _ _ _ _ _ _ _ _ _ _ _ _ _ w548 w555]
      tunnel: w365 -> [_ _ _ _ _ _ _ _ _ _ _ _ _ _ w481 _ _ _ _ _ _ _ _ _ _ _]
      tunnel: w364 -> [_ _ _ _ _ _ _ _ _ _ _ _ _ w477 _ _ _ _ _ _ _ _ _ _ _ _]
      event Timeout {
        n202 = event-data() -> ()  [unwired: 1 in, 3 out]
      }
      event "校准": Value Change {
        n203 = event-data() -> ()  [unwired: 1 in, 6 out]
        n204 = call "校准画面.vi"() -> ()  [unwired: 12 in]
      }
      event "K", "B", "水深校准", "水样稳定时间", "上电初始化时间", "转刷清洗时间", "水样测试组数", "标样测试组数": Mouse Down {
        n205 = event-data() -> ("CtlRef"=w372:refnum<vi>)  [unwired: 1 in, 7 out]
        n206 = property class="DigNum (严格)"(reference=w372) -> (reference out=w370:refnum<vi>, "Value"=w371:dbl)  [unwired: 1 in, 1 out]
        n207 = call "数字键盘.vi"("OldNumber"=w371) -> ("NewNumber"=w369:dbl)
        n208 = property class="DigNum (严格)"(reference=w370, "Value"=w369) -> ()  [unwired: 1 in, 2 out]
      }
      event "读取": Value Change {
        n209 = event-data() -> ()  [unwired: 1 in, 6 out]
        n210 = property class="Ring (严格)"(reference=w376) -> ("Value"=w375:u16)  [unwired: 1 in, 2 out]
        n211 = call "多参校准读取.vi"("站号"=w375) -> ("B"=w373:dbl, "K"=w374:dbl)  [unwired: 8 in, 1 out]
        n212 = local write "K"(w374) -> ()
        n213 = local write "B"(w373) -> ()
      }
      event "写入": Value Change {
        n214 = event-data() -> ()  [unwired: 1 in, 6 out]
        n215 = property class="Ring (严格)"(reference=w380) -> ("Value"=w379:u16)  [unwired: 1 in, 2 out]
        n216 = call "多参数校准写入.vi"("B"="B", "K"="K", "站号"=w379) -> ()  [unwired: 8 in, 1 out]
      }
      event "水深读取": Value Change {
        w382 = u16 9 items=["氨氮"=3, "水温"=9, "pH值"=10, "溶解氧"=11, "电导率"=12, "浊度"=13, "叶绿素a"=14, "藻密度"=15, "蓝绿藻"=16, "氧化还原电位"=17, "溶解氧%"=18, "盐度"=19] ("站号")
        n217 = event-data() -> ()  [unwired: 1 in, 6 out]
        n218 = call "多参水深校准读取.vi"("站号"=w382) -> ("B"=w381:dbl)  [unwired: 8 in, 2 out]
        n219 = local write "水深校准"(w381) -> ()
      }
      event "水深写入": Value Change {
        w384 = u16 9 items=["氨氮"=3, "水温"=9, "pH值"=10, "溶解氧"=11, "电导率"=12, "浊度"=13, "叶绿素a"=14, "藻密度"=15, "蓝绿藻"=16, "氧化还原电位"=17, "溶解氧%"=18, "盐度"=19] ("站号")
        n220 = event-data() -> ()  [unwired: 1 in, 6 out]
        n221 = call "多参数水深校准写入.vi"("K"="水深校准", "站号"=w384) -> ()  [unwired: 9 in, 1 out]
      }
      event "串口设置": Value Change {
        n222 = event-data() -> ()  [unwired: 1 in, 6 out]
        n223 = global read "多参数断电保存全局变量.vi" "VISA Resource"() -> (w389:refnum<visa-resource-name>)
        n224 = global read "多参数断电保存全局变量.vi" "波特率"() -> (w387:u32)
        n225 = call "串口配置.vi"("波特率"=w387, "VISA资源名称"=w389) -> ("确认 2"=w385:bool, "波特率 2"=w386:u32, "VISA资源名称 2"=w388:refnum<visa-resource-name>)  [unwired: 7 in]
        n226 = case shown="真" w385 {
          tunnel: w388 -> [_ w391]
          tunnel: w386 -> [_ w390]
          frame False {
          }
          frame True {
            n227 = flat-sequence {
              tunnel: w391 -> [w393]
              tunnel: w390 -> [w392]
              frame #0 {
                n228 = global write "多参数断电保存全局变量.vi" "VISA Resource"(w393) -> ()
                n229 = global write "多参数断电保存全局变量.vi" "波特率"(w392) -> ()
              }
              frame #1 {
                n230 = call "多参数通讯.vi"("STEP"=enum16{"open", "read", "write", "close"}."open") -> ("error out"=w395:errorcluster)  [unwired: 8 in, 2 out]
                n231 = case shown="错误" w395 {
                  frame No Error {
                  }
                  frame Error {
                    n232 = One Button Dialog(message="多参数串口打开失败" ("消息")) -> ()  [unwired: 1 in, 1 out]
                  }
                }
              }
              frame #2 {
                n233 = call <vilib>:"Application Directory.vi"() -> ("Application Directory"=w410:path)
                n234 = Build Path(base path=w410, name or relative path="data\\sys.ini" ("名称或相对路径")) -> (appended path=w408:path)
                n235 = call <vilib>:"Open Config Data.vi"("configuration file path"=w408) -> ("error out"=w404:errorcluster, "refnum"=w407:T11)  [unwired: 8 in, 1 out]
                n236 = vi-ref "多参数断电保存全局变量.vi"() -> (w406:refnum<vi>)
                n237 = call <userlib>:"Write Panel to INI__ogtk.vi"("error in (no error)"=w404, "VI ref"=w406, "refnum"=w407) -> ("error out"=w403:errorcluster, "refnum out"=w405:T11)  [unwired: 7 in]
                n238 = call <vilib>:"Close Config Data.vi"("error in (no error)"=w403, "refnum"=w405) -> ("error out"=w398:errorcluster, "file path"=w397:path)  [unwired: 8 in]
                n239 = Open/Create/Replace File(file path (use dialog)=w397, error in=w398) -> (refnum out=w401:refnum<file>, error out=w402:errorcluster)  [unwired: 4 in, 1 out]
                n240 = Flush File(refnum=w401, error in=w402) -> (refnum out=w400:refnum<file>, error out=w399:errorcluster)
                n241 = Close File(refnum=w400, error in=w399) -> ()  [unwired: 2 out]
              }
            }
          }
        }
      }
      event "水样稳定时间", "上电初始化时间", "转刷清洗时间", "水样测试组数", "标样测试组数": Value Change {
        n242 = event-data() -> ()  [unwired: 1 in, 6 out]
        n243 = flat-sequence {
          frame #0 {
            n244 = global write "多参数断电保存全局变量.vi" "水样稳定时间"("水样稳定时间") -> ()
            n245 = global write "多参数断电保存全局变量.vi" "水样测试组数"("水样测试组数") -> ()
            n246 = global write "多参数断电保存全局变量.vi" "上电初始化时间"("上电初始化时间") -> ()
            n247 = global write "多参数断电保存全局变量.vi" "转刷清洗时间"("转刷清洗时间") -> ()
            n248 = global write "多参数断电保存全局变量.vi" "标样测试组数"("标样测试组数") -> ()
          }
          frame #1 {
            n249 = call "配置保存.vi"() -> ()  [unwired: 11 in, 1 out]
          }
        }
      }
      event "传感器参数自动获取": Value Change {
        n250 = event-data() -> ("NewVal"=w416:bool)  [unwired: 1 in, 5 out]
        n251 = case shown="假" w416 {
          frame False {
            n252 = property on="获取传感器参数并保存触发" class="Bool (严格)"("Val(Sgnl)"=FALSE ("获取传感器参数并保存触发")) -> ()  [unwired: 2 in, 2 out]
          }
          frame True {
          }
        }
        n253 = flat-sequence {
          tunnel: w416 -> [w418]
          frame #0 {
            n254 = global write "多参数断电保存全局变量.vi" "传感器参数自动获取"(w418) -> ()
          }
          frame #1 {
            n255 = call <vilib>:"Application Directory.vi"() -> ("Application Directory"=w432:path)
            n256 = Build Path(base path=w432, name or relative path="data\\sys.ini" ("名称或相对路径")) -> (appended path=w430:path)
            n257 = call <vilib>:"Open Config Data.vi"("configuration file path"=w430) -> ("error out"=w426:errorcluster, "refnum"=w429:T11)  [unwired: 8 in, 1 out]
            n258 = vi-ref "多参数断电保存全局变量.vi"() -> (w428:refnum<vi>)
            n259 = call <userlib>:"Write Panel to INI__ogtk.vi"("error in (no error)"=w426, "VI ref"=w428, "refnum"=w429) -> ("error out"=w425:errorcluster, "refnum out"=w427:T11)  [unwired: 7 in]
            n260 = call <vilib>:"Close Config Data.vi"("error in (no error)"=w425, "refnum"=w427) -> ("error out"=w420:errorcluster, "file path"=w419:path)  [unwired: 8 in]
            n261 = Open/Create/Replace File(file path (use dialog)=w419, error in=w420) -> (refnum out=w423:refnum<file>, error out=w424:errorcluster)  [unwired: 4 in, 1 out]
            n262 = Flush File(refnum=w423, error in=w424) -> (refnum out=w422:refnum<file>, error out=w421:errorcluster)
            n263 = Close File(refnum=w422, error in=w421) -> ()  [unwired: 2 out]
          }
        }
      }
      event "质控参数设置": Value Change {
        n264 = event-data() -> ()  [unwired: 1 in, 6 out]
        n265 = global read "多参数断电保存全局变量.vi" "质控参数设置"() -> (w433:T12)
        n266 = call "多参数质控参数设置.vi"("质控参数设置"=w433) -> ("输出簇"=w434:T13)  [unwired: 10 in]
        n267 = Unbundle By Name(w434) -> ("确定"=w435:bool)
        n268 = case shown="真" w435 {
          tunnel: w434 -> [_ w437]
          tunnel: w433 -> [_ w436]
          frame False {
          }
          frame True {
            n269 = flat-sequence {
              tunnel: w437 -> [w445]
              tunnel: w436 -> [w444]
              frame #0 {
                n270 = Unbundle By Name(w445) -> ("水温标准液标准浓度"=w443:dbl, "酸碱度标准液标准浓度"=w442:dbl, "溶解氧标准液标准浓度"=w441:dbl, "电导率标准液标准浓度"=w440:dbl, "浊度标准液标准浓度"=w439:dbl)
                n271 = Bundle By Name(cluster=w444, "水温标准液标准浓度"=w443, "酸碱度标准液标准浓度"=w442, "溶解氧标准液标准浓度"=w441, "电导率标准液标准浓度"=w440, "浊度标准液标准浓度"=w439) -> (w438:T12)
                n272 = global write "多参数断电保存全局变量.vi" "质控参数设置"(w438) -> ()
              }
              frame #1 {
                n273 = call <vilib>:"Application Directory.vi"() -> ("Application Directory"=w459:path)
                n274 = Build Path(base path=w459, name or relative path="data\\sys.ini" ("名称或相对路径")) -> (appended path=w457:path)
                n275 = call <vilib>:"Open Config Data.vi"("configuration file path"=w457) -> ("error out"=w453:errorcluster, "refnum"=w456:T11)  [unwired: 8 in, 1 out]
                n276 = vi-ref "多参数断电保存全局变量.vi"() -> (w455:refnum<vi>)
                n277 = call <userlib>:"Write Panel to INI__ogtk.vi"("error in (no error)"=w453, "VI ref"=w455, "refnum"=w456) -> ("error out"=w452:errorcluster, "refnum out"=w454:T11)  [unwired: 7 in]
                n278 = call <vilib>:"Close Config Data.vi"("error in (no error)"=w452, "refnum"=w454) -> ("error out"=w447:errorcluster, "file path"=w446:path)  [unwired: 8 in]
                n279 = Open/Create/Replace File(file path (use dialog)=w446, error in=w447) -> (refnum out=w450:refnum<file>, error out=w451:errorcluster)  [unwired: 4 in, 1 out]
                n280 = Flush File(refnum=w450, error in=w451) -> (refnum out=w449:refnum<file>, error out=w448:errorcluster)
                n281 = Close File(refnum=w449, error in=w448) -> ()  [unwired: 2 out]
              }
            }
          }
        }
      }
      event "释放串口": Value Change {
        n282 = event-data() -> ("NewVal"=w460:bool)  [unwired: 1 in, 5 out]
        n283 = case shown="真" w460 {
          frame False {
          }
          frame True {
            n284 = call "多参数通讯.vi"("STEP"=enum16{"open", "read", "write", "close"}."close") -> ("error out"=w461:errorcluster)  [unwired: 8 in, 2 out]
            n285 = case shown="无错误" w461 {
              frame No Error {
                n286 = property on="打开串口" class="Bool (严格)"("DisabledEnum"=T8."Enabled" ("禁用")) -> ()  [unwired: 2 in, 2 out]
              }
              frame Error {
              }
            }
          }
        }
      }
      event "打开串口": Value Change {
        n287 = event-data() -> ("NewVal"=w464:bool)  [unwired: 1 in, 5 out]
        n288 = case shown="真" w464 {
          frame False {
          }
          frame True {
            n289 = call "多参数通讯.vi"("STEP"=enum16{"open", "read", "write", "close"}."open") -> ("error out"=w465:errorcluster)  [unwired: 8 in, 2 out]
            n290 = case shown="错误" w465 {
              tunnel: [T8."Disabled and Grayed Out" ("禁用") T8."Enabled" ("禁用")] -> w467
              frame No Error {
              }
              frame Error {
                n291 = One Button Dialog(message="多参数串口打开失败" ("消息")) -> ()  [unwired: 1 in, 1 out]
              }
            }
            n292 = property on="打开串口" class="Bool (严格)"("DisabledEnum"=w467, "Value"=FALSE ("打开串口")) -> ()  [unwired: 2 in, 2 out]
          }
        }
      }
      event "水样测试": Value Change {
        n293 = event-data() -> ()  [unwired: 1 in, 6 out]
        n294 = global read "多参数断电保存全局变量.vi" "运行周期"() -> (w475:T14)
        n295 = Unbundle By Name(w475) -> ("运行模式"=w474:enum16{"维护模式", "常规模式", "应急模式", "质控模式"})
        n296 = case shown="\"维护模式\"" w474 {
          tunnel: ["M" ("数据类型") "hd" ("数据类型")] -> w472
          frame "维护模式" {
          }
          frame "常规模式", Default {
          }
        }
        n297 = Bundle By Name(cluster=T9 {"测量模式"="水样测试", "数据类型"="N"} ("启动参数"), "数据类型"=w472) -> (w473:T9)
        n298 = Enqueue Element(queue=w477, element=w473) -> ()  [unwired: 2 in, 3 out]
      }
      event "标样核查": Value Change {
        n299 = event-data() -> ()  [unwired: 1 in, 6 out]
        n300 = call "多参数标样核查对话框.vi"() -> ("确认"=w482:bool, "输出参数"=w480:T15)  [unwired: 10 in]
        n301 = case shown="真" w482 {
          tunnel: w481 -> [_ w485]
          tunnel: w480 -> [_ w484]
          frame False {
          }
          frame True {
            n302 = property class="VI"(reference=w485) -> ("Name"=w489:string, "Exec.State"=w487:T16)  [unwired: 1 in, 2 out]
            n303 = Open VI Reference(type specifier VI Refnum (for type only)=refnum<vi> refnum, vi path=w489, options=128 ("选项")) -> (vi reference=w488:refnum<vi>)  [unwired: 3 in, 1 out]
            n304 = case shown="\"Idle\"" w487 {
              tunnel: w488 -> [w492 w500]
              tunnel: [w492 w499] -> w486
              tunnel: w484 -> [_ w497]
              frame "Bad", Default {
                n305 = One Button Dialog(message="仪器已经启动，无需重复启动" ("消息")) -> ()  [unwired: 1 in, 1 out]
              }
              frame "Idle" {
                n306 = global read "多参数断电保存全局变量.vi" "运行周期"() -> (w496:T14)
                n307 = Unbundle By Name(w496) -> ("运行模式"=w495:enum16{"维护模式", "常规模式", "应急模式", "质控模式"})
                n308 = case shown="\"维护模式\"" w495 {
                  tunnel: ["M" ("数据标记表") "N" ("数据标记表")] -> w498
                  frame "维护模式" {
                  }
                  frame "常规模式", Default {
                  }
                }
                n309 = Bundle By Name(cluster=T10 {"测量模式"="标样核查", "数据类型"="N", "输出参数"={"水温"=FALSE, "pH"=FALSE, "DO"=FALSE, "浊度"=FALSE, "电导率"=FALSE}} ("启动参数"), "数据类型"=w498, "输出参数"=w497) -> (w493:T10)
                n310 = call-by-ref "开始异步调用"(reference=w500, "启动参数"=w493) -> (reference out=w499:refnum<vi>)  [unwired: 12 in, 1 out]
              }
            }
            n311 = Close Reference(reference=w486) -> ()  [unwired: 1 in, 1 out]
          }
        }
      }
      event "停止": Value Change {
        n312 = event-data() -> ()  [unwired: 1 in, 6 out]
        n313 = Two Button Dialog(message="请再一次确认是否停止测量" ("消息")) -> (T button?=w503:bool)  [unwired: 2 in]
        n314 = case shown="真" w503 {
          tunnel: w505 -> [_ w508]
          frame False {
          }
          frame True {
            w506 = u16 11 items=["启动测量（全部）"=1, "初始化（清洗）"=10, "停止测量（全部）"=11, "校时"=13, "启动测量（单个传感器）"=19, "停止测量（单个传感器）"=20] ("控制命令")
            w507 = u16 10 items=["氨氮"=3, "水温"=9, "pH值"=10, "溶解氧"=11, "电导率"=12, "浊度"=13, "叶绿素a"=14, "藻密度"=15, "蓝绿藻"=16, "氧化还原电位"=17, "溶解氧%"=18, "盐度"=19] ("站号")
            n315 = Send Notification(notification=TRUE ("通知"), notifier=w508) -> ()  [unwired: 1 in, 2 out]
            n316 = call "多参数控制命令.vi"("控制命令"=w506, "站号"=w507) -> ()  [unwired: 9 in, 1 out]
          }
        }
      }
      event "设置": Value Change {
        n317 = event-data() -> ()  [unwired: 1 in, 6 out]
        n318 = property on="窗格" class="Pane"("Origin"=T2 {"Horizontal"=0, "Vertical"=628} ("原点")) -> ()  [unwired: 2 in, 2 out]
      }
      event "返回": Value Change {
        n319 = event-data() -> ()  [unwired: 1 in, 6 out]
        n320 = property on="窗格" class="Pane"("Origin"=T2 {"Horizontal"=0, "Vertical"=0} ("原点")) -> ()  [unwired: 2 in, 2 out]
      }
      event "传感器参数读取", "获取传感器参数并保存触发": Value Change {
        n321 = event-data() -> ()  [unwired: 1 in, 6 out]
        n322 = call "多参数传感器参数读取.vi"() -> ("error out"=w515:errorcluster, "modbus"=w513:u16[], "添加的数组"=w514:string[][])  [unwired: 9 in]
        n323 = property on="传感器区" class="MCListbox (严格)"("ItemNames"=w514) -> ()  [unwired: 2 in, 2 out]
        n324 = call <vilib>:"General Error Handler.vi"("error in (no error)"=w515) -> ("error out"=w512:errorcluster)  [unwired: 10 in, 4 out]
        n325 = case shown="无错误" w512 {
          tunnel: w513 -> [w516 _]
          frame No Error {
            n326 = flat-sequence {
              tunnel: w516 -> [w517]
              frame #0 {
                n327 = global write "多参数断电保存全局变量.vi" "传感器参数modbus"(w517) -> ()
              }
              frame #1 {
                n328 = call "配置保存.vi"() -> ()  [unwired: 11 in, 1 out]
              }
            }
          }
          frame Error {
          }
        }
      }
      event "关键参数区读取": Value Change {
        n329 = event-data() -> ()  [unwired: 1 in, 6 out]
        n330 = call "多参数关键参数读取.vi"() -> ("error out"=w518:errorcluster, "添加的数组"=w519:string[][])  [unwired: 10 in]
        n331 = property on="关键参数区" class="MCListbox (严格)"("ItemNames"=w519) -> ()  [unwired: 2 in, 2 out]
        n332 = call <vilib>:"General Error Handler.vi"("error in (no error)"=w518) -> ()  [unwired: 10 in, 5 out]
      }
      event "同步时间": Value Change {
        w520 = u16 13 items=["启动测量（全部）"=1, "初始化（清洗）"=10, "停止测量（全部）"=11, "校时"=13, "启动测量（单个传感器）"=19, "停止测量（单个传感器）"=20] ("控制命令")
        w521 = u16 9 items=["氨氮"=3, "水温"=9, "pH值"=10, "溶解氧"=11, "电导率"=12, "浊度"=13, "叶绿素a"=14, "藻密度"=15, "蓝绿藻"=16, "氧化还原电位"=17, "溶解氧%"=18, "盐度"=19] ("站号")
        n333 = event-data() -> ()  [unwired: 1 in, 6 out]
        n334 = call "多参数控制命令.vi"("控制命令"=w520, "站号"=w521) -> ("error out"=w523:errorcluster)  [unwired: 9 in]
        n335 = case shown="错误" w523 {
          tunnel: ["时间同步成功" ("消息") "时间同步失败" ("消息")] -> w522
          frame No Error {
          }
          frame Error {
          }
        }
        n336 = One Button Dialog(message=w522) -> ()  [unwired: 1 in, 1 out]
      }
      event "启动测量(全部)": Value Change {
        w526 = u16 1 items=["启动测量（全部）"=1, "初始化（清洗）"=10, "停止测量（全部）"=11, "校时"=13, "启动测量（单个传感器）"=19, "停止测量（单个传感器）"=20] ("控制命令")
        w527 = u16 9 items=["氨氮"=3, "水温"=9, "pH值"=10, "溶解氧"=11, "电导率"=12, "浊度"=13, "叶绿素a"=14, "藻密度"=15, "蓝绿藻"=16, "氧化还原电位"=17, "溶解氧%"=18, "盐度"=19] ("站号")
        n337 = event-data() -> ()  [unwired: 1 in, 6 out]
        n338 = call "多参数控制命令.vi"("控制命令"=w526, "站号"=w527) -> ("error out"=w529:errorcluster)  [unwired: 9 in]
        n339 = case shown="无错误" w529 {
          tunnel: ["启动成功" ("消息") "启动失败" ("消息")] -> w528
          frame No Error {
          }
          frame Error {
          }
        }
        n340 = One Button Dialog(message=w528) -> ()  [unwired: 1 in, 1 out]
      }
      event "停止测量(全部)": Value Change {
        w534 = u16 11 items=["启动测量（全部）"=1, "初始化（清洗）"=10, "停止测量（全部）"=11, "校时"=13, "启动测量（单个传感器）"=19, "停止测量（单个传感器）"=20] ("控制命令")
        w535 = u16 9 items=["氨氮"=3, "水温"=9, "pH值"=10, "溶解氧"=11, "电导率"=12, "浊度"=13, "叶绿素a"=14, "藻密度"=15, "蓝绿藻"=16, "氧化还原电位"=17, "溶解氧%"=18, "盐度"=19] ("站号")
        n341 = event-data() -> ()  [unwired: 1 in, 6 out]
        n342 = call "多参数控制命令.vi"("控制命令"=w534, "站号"=w535) -> ("error out"=w533:errorcluster)  [unwired: 9 in]
        n343 = case shown="错误" w533 {
          tunnel: ["停止成功" ("消息") "停止失败" ("消息")] -> w532
          frame No Error {
          }
          frame Error {
          }
        }
        n344 = One Button Dialog(message=w532) -> ()  [unwired: 1 in, 1 out]
      }
      event "初始化(清洗)": Value Change {
        w540 = u16 10 items=["启动测量（全部）"=1, "初始化（清洗）"=10, "停止测量（全部）"=11, "校时"=13, "启动测量（单个传感器）"=19, "停止测量（单个传感器）"=20] ("控制命令")
        w541 = u16 9 items=["氨氮"=3, "水温"=9, "pH值"=10, "溶解氧"=11, "电导率"=12, "浊度"=13, "叶绿素a"=14, "藻密度"=15, "蓝绿藻"=16, "氧化还原电位"=17, "溶解氧%"=18, "盐度"=19] ("站号")
        n345 = event-data() -> ()  [unwired: 1 in, 6 out]
        n346 = call "多参数控制命令.vi"("控制命令"=w540, "站号"=w541) -> ("error out"=w538:errorcluster)  [unwired: 9 in]
        n347 = case shown="错误" w538 {
          tunnel: ["初始化成功" ("消息") "初始化失败" ("消息")] -> w539
          frame No Error {
          }
          frame Error {
          }
        }
        n348 = One Button Dialog(message=w539) -> ()  [unwired: 1 in, 1 out]
      }
      event "启动测量(单探)": Value Change {
        w544 = u16 19 items=["启动测量（全部）"=1, "初始化（清洗）"=10, "停止测量（全部）"=11, "校时"=13, "启动测量（单个传感器）"=19, "停止测量（单个传感器）"=20] ("控制命令")
        n349 = event-data() -> ()  [unwired: 1 in, 6 out]
        n350 = property class="Ring (严格)"(reference=w548) -> ("Value"=w547:u16)  [unwired: 1 in, 2 out]
        n351 = call "多参数控制命令.vi"("控制命令"=w544, "站号"=w547) -> ("error out"=w546:errorcluster)  [unwired: 9 in]
        n352 = case shown="无错误" w546 {
          tunnel: ["启动成功" ("消息") "启动失败" ("消息")] -> w545
          frame No Error {
          }
          frame Error {
          }
        }
        n353 = One Button Dialog(message=w545) -> ()  [unwired: 1 in, 1 out]
      }
      event "停止测量(单探)": Value Change {
        w551 = u16 20 items=["启动测量（全部）"=1, "初始化（清洗）"=10, "停止测量（全部）"=11, "校时"=13, "启动测量（单个传感器）"=19, "停止测量（单个传感器）"=20] ("控制命令")
        n354 = event-data() -> ()  [unwired: 1 in, 6 out]
        n355 = property class="Ring (严格)"(reference=w555) -> ("Value"=w554:u16)  [unwired: 1 in, 2 out]
        n356 = call "多参数控制命令.vi"("控制命令"=w551, "站号"=w554) -> ("error out"=w553:errorcluster)  [unwired: 9 in]
        n357 = case shown="错误" w553 {
          tunnel: ["停止成功" ("消息") "停止失败" ("消息")] -> w552
          frame No Error {
          }
          frame Error {
          }
        }
        n358 = One Button Dialog(message=w552) -> ()  [unwired: 1 in, 1 out]
      }
    }
  }
